vi "Naleeya's Quiz Course.vi"() -> ()   [LabVIEW 2018]
panel:
  out "Coolness Bar":u8(slide) scale=0.0..100.0
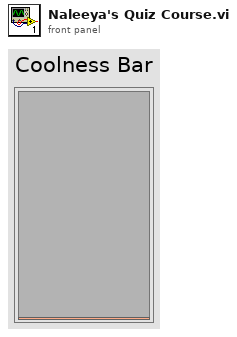
[diagram p1: front panel]
types:
  T1 = enum16{"Left Button", "Center Button", "Right Button", "Window Close"}
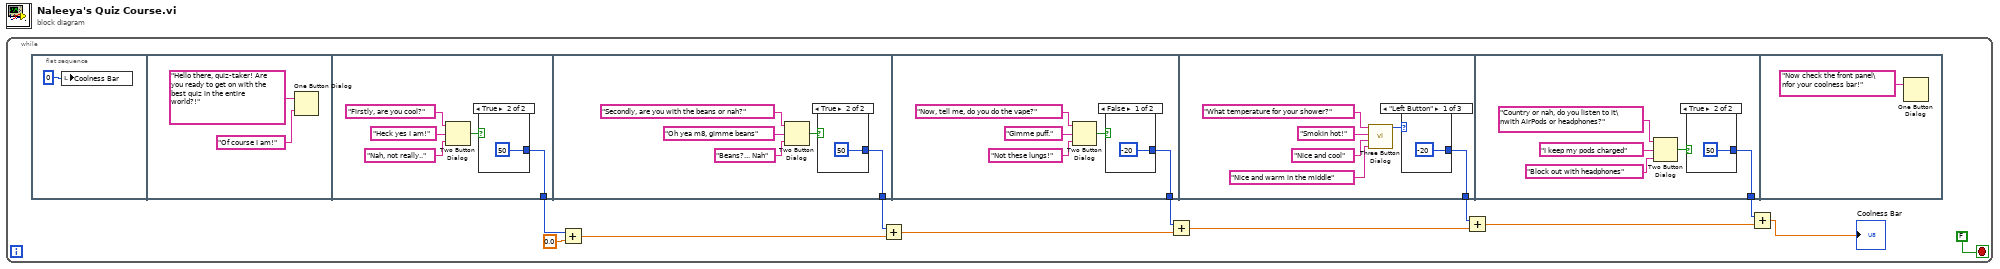
[diagram p0: block diagram]
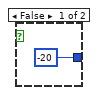
[diagram p2: hidden frame]
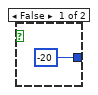
[diagram p3: hidden frame]
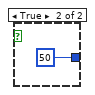
[diagram p4: hidden frame]
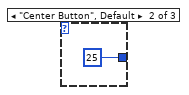
[diagram p5: hidden frame]
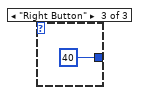
[diagram p6: hidden frame]
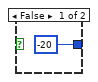
[diagram p7: hidden frame]
diagram:
  n1 = while {
    stop <- FALSE stop-if-true
    n2 = flat-sequence {
      tunnel: [w20] -> w10
      tunnel: [w23] -> w8
      tunnel: [w30] -> w6
      tunnel: [w37] -> w4
      tunnel: [w48] -> w2
      frame #0 {
        n3 = local write "Coolness Bar"(u8 0 ("Coolness Bar")) -> ()
      }
      frame #1 {
        n4 = One Button Dialog(message="Hello there, quiz-taker! Are you ready to get on with the best quiz in the entire world?!", button name ("OK")="Of course I am!") -> ()  [unwired: 1 out]
      }
      frame #2 {
        n5 = Two Button Dialog(message="Firstly, are you cool?", 1:"Nah, not really.." ("F button name (\"Cancel\")"), 2:"Heck yes I am!" ("T button name (\"OK\")")) -> (T button?=w16:bool)
        n6 = case shown="True" w16 {
          tunnel: [-20 50] -> w20
          frame False {
          }
          frame True {
          }
        }
      }
      frame #3 {
        n7 = Two Button Dialog(message="Secondly, are you with the beans or nah?", 1:"Beans?... Nah" ("F button name (\"Cancel\")"), 2:"Oh yea m8, gimme beans" ("T button name (\"OK\")")) -> (T button?=w24:bool)
        n8 = case shown="True" w24 {
          tunnel: [-20 50] -> w23
          frame False {
          }
          frame True {
          }
        }
      }
      frame #4 {
        n9 = Two Button Dialog(message="Now, tell me, do you do the vape?", 1:"Not these lungs!" ("F button name (\"Cancel\")"), 2:"Gimme puff." ("T button name (\"OK\")")) -> (T button?=w31:bool)
        n10 = case shown="False" w31 {
          tunnel: [-20 50] -> w30
          frame False {
          }
          frame True {
          }
        }
      }
      frame #5 {
        n11 = call <vilib>:"Three Button Dialog.vi"("Right Button Text (\"Cancel\")"="Nice and warm in the middle" ("Right Button Text (\"Cancel\")"), "Center Button Text (\"No\")"="Nice and cool" ("F button name (\"Cancel\")"), "Left Button Text (\"Yes\")"="Smokin hot!" ("T button name (\"OK\")"), "message"="What temperature for your shower?") -> ("Which Button?"=w42:T1)  [unwired: 7 in]
        n12 = case shown="\"Left Button\"" w42 {
          tunnel: [-20 25 40] -> w37
          frame "Left Button" {
          }
          frame "Center Button", Default {
          }
          frame "Right Button" {
          }
        }
      }
      frame #6 {
        n13 = Two Button Dialog(message="Country or nah, do you listen to it\nwith AirPods or headphones?", 1:"Block out with headphones" ("F button name (\"Cancel\")"), 2:"I keep my pods charged" ("T button name (\"OK\")")) -> (T button?=w49:bool)
        n14 = case shown="True" w49 {
          tunnel: [-20 50] -> w48
          frame False {
          }
          frame True {
          }
        }
      }
      frame #7 {
        n15 = One Button Dialog(message="Now check the front panel\nfor your coolness bar!") -> ()  [unwired: 1 in, 1 out]
      }
    }
    n16 = Add(x=w10, y=0.0) -> (x+y=w9:dbl)
    n17 = Add(x=w8, y=w9) -> (x+y=w7:dbl)
    n18 = Add(x=w6, y=w7) -> (x+y=w5:dbl)
    n19 = Add(x=w4, y=w5) -> (x+y=w3:dbl)
    n20 = Add(x=w2, y=w3) -> (x+y=→"Coolness Bar":dbl)
  }
